vi "PSDATA_Variant To ArrayStr.vi"(9 "error in":errorcluster, 10 "Value":variant) -> (1 "error out":errorcluster, 2 "Value":string, 4 "ArrayStr":string[](array[string]))   [LabVIEW 2016]
doc: "Developer：YDX"
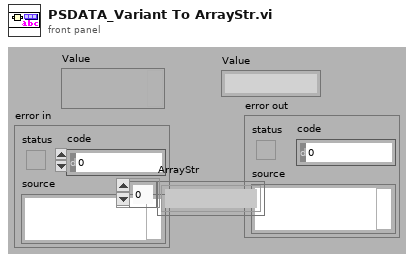
[diagram p1: front panel]
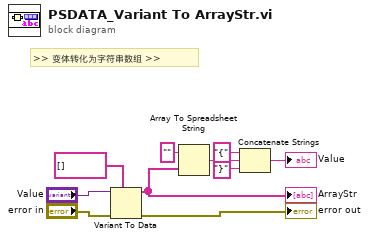
[diagram p0: block diagram]
diagram:
  # ">> 变体转化为字符串数组 >>"
  n1 = Variant To Data(error in="error in", type=string[] [], Variant="Value") -> (data=w1:string[], error out=→"error out":errorcluster)
  "ArrayStr" <- w1
  n2 = Array To Spreadsheet String(array=w1, 3:"" ("format string")) -> (spreadsheet string=w6:string)  [unwired: 1 in]
  n3 = Concatenate Strings("{" ("string"), w6, "}" ("string")) -> (→"Value":string)
